vi "MIME TIFF Parser.vi"() -> ()   [LabVIEW 2014]
panel:
  out "Cluster":T1
  in  "Path":path
  out "Decompress":bool
  out "data out":string
  out "Width":u32
  out "Height":u32
  in  "error in (no error)":errorcluster
  out "error out":errorcluster
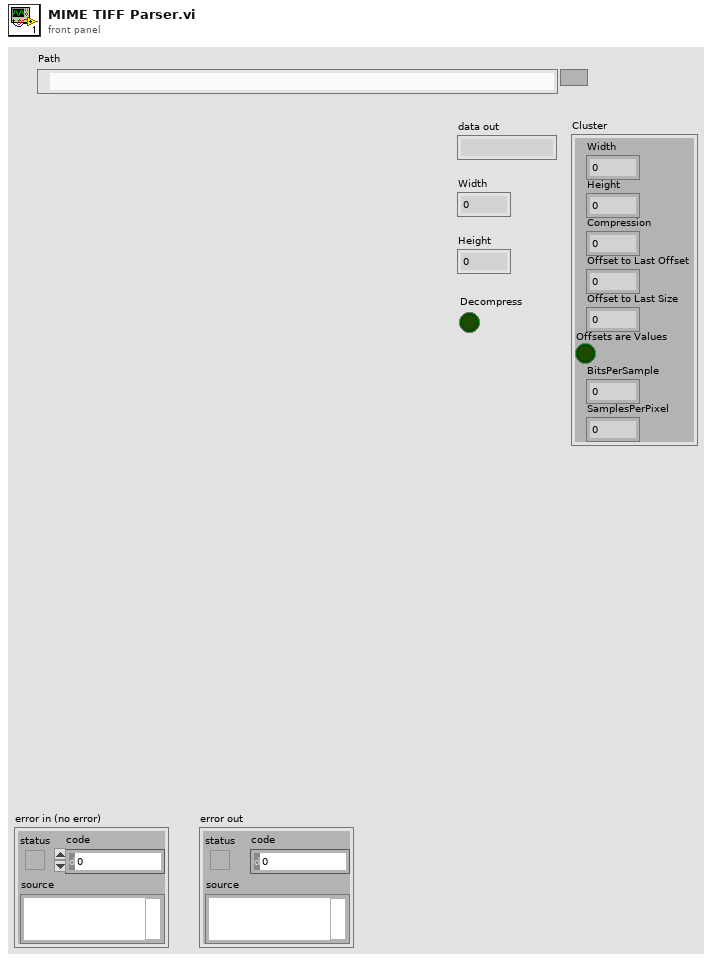
[diagram p1: front panel]
types:
  T1 = cluster{"Width":u32, "Height":u32, "Compression":u32, "Offset to Last Offset":u32, "Offset to Last Size":u32, "Offsets are Values":bool, "BitsPerSample":u32, "SamplesPerPixel":u32}
  T2 = cluster{"Tag":u16, "Type":enum16{"NONE", "Byte", "ASCII", "Short", "Long", "Rational", "SByte", "Undefined", "SShort", "SLong", "SRational", "Float", "Double"}, "Count":u32, "Value/Offset":u32}
  T3 = enum16{"big-endian, network order", "native, host order", "little-endian"}
  T4 = cluster{"Tag":u16, "Type":enum16{"NONE", "Byte", "ASCII", "Short", "Long", "Rational", "SByte", "Undefined", "SShort", "SLong", "SRational", "Float", "Double"}, "Count":u32, "Value/Offset":u32}[]
  T5 = enum16{"NONE", "Byte", "ASCII", "Short", "Long", "Rational", "SByte", "Undefined", "SShort", "SLong", "SRational", "Float", "Double"}
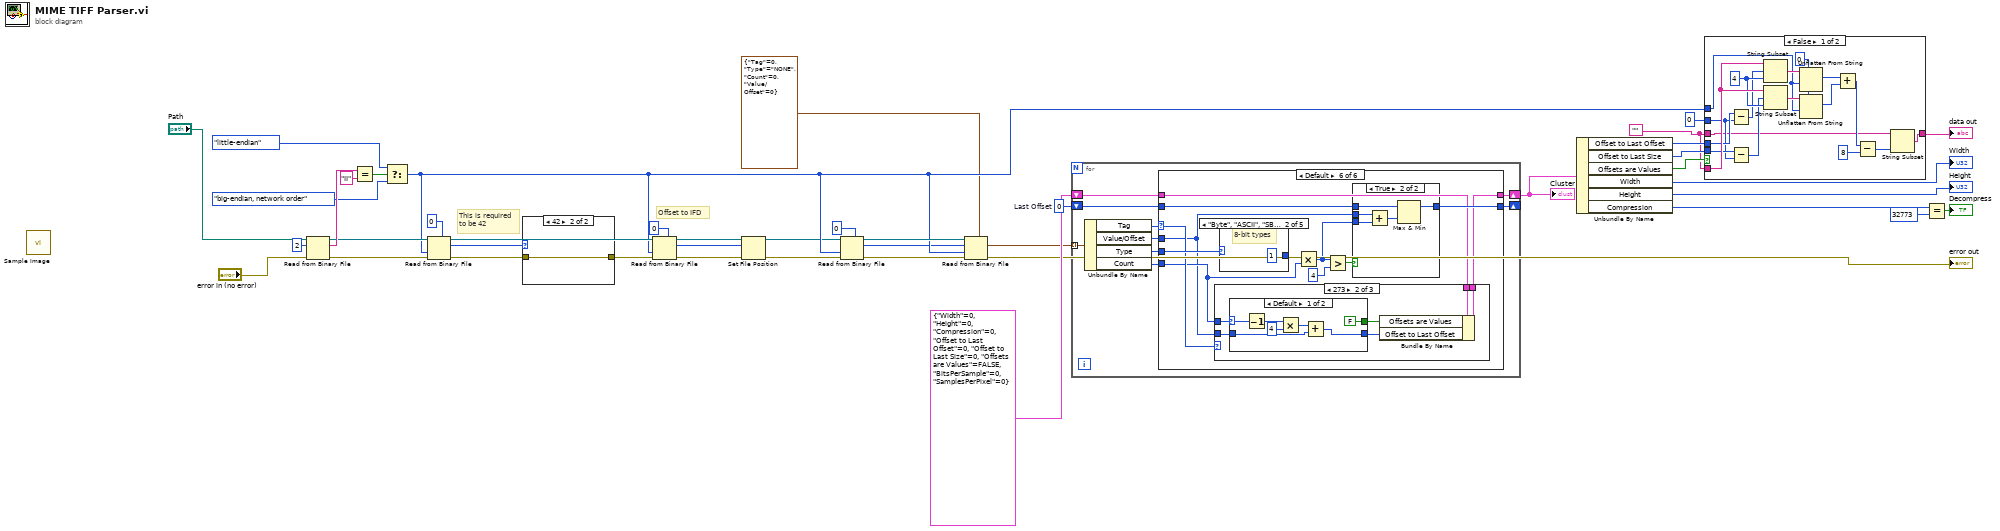
[diagram p0: block diagram]
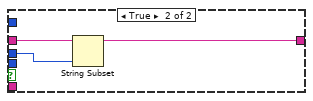
[diagram p2: hidden frame]
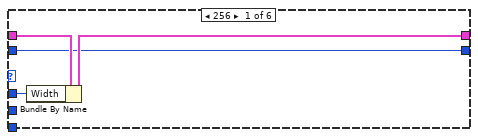
[diagram p3: hidden frame]
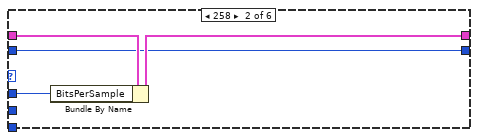
[diagram p4: hidden frame]
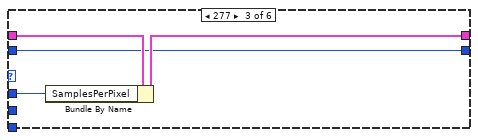
[diagram p5: hidden frame]
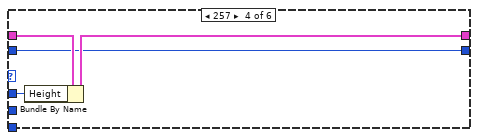
[diagram p6: hidden frame]
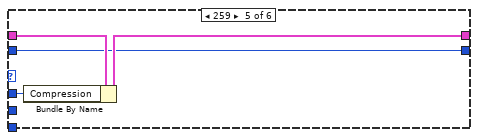
[diagram p7: hidden frame]
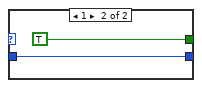
[diagram p9: hidden frame]
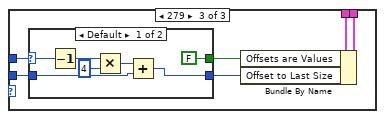
[diagram p10: hidden frame]
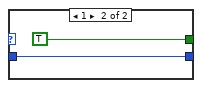
[diagram p11: hidden frame]
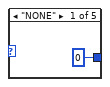
[diagram p13: hidden frame]
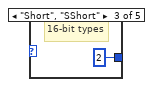
[diagram p14: hidden frame]
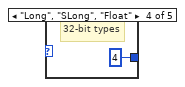
[diagram p15: hidden frame]
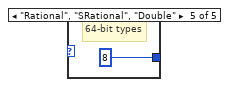
[diagram p16: hidden frame]
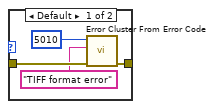
[diagram p17: hidden frame]
diagram:
  w1 = ""
  w36 = u32 0  # Last Offset
  # "Offset to IFD"
  # "This is required\nto be 42"
  n1 = call "Sample Image.vi"() -> ()  [unwired: 11 in, 1 out]
  n2 = Read from Binary File(8:"error in (no error)", 10:2 ("bytes to read"), 11:"Path") -> (0:w27:errorcluster, 2:w25:string, 3:w22:refnum<file>)  [unwired: 3 in, 1 out]
  n3 = Equal?(x=w25, y="II") -> (x = y?=w41:bool)
  n4 = Select(t=T3."little-endian" ("byte order (0:big-endian, network order)"), s=w41, f=T3."big-endian, network order" ("byte order (0:big-endian, network order)")) -> (s? t:f=w15:T3)
  n5 = Read from Binary File(5:u16 0, 8:w27, 9:w15, 11:w22) -> (0:w20:errorcluster, 2:w19:u16, 3:w43:refnum<file>)  [unwired: 2 in, 1 out]
  n6 = case shown="42" w19 {
    tunnel: w20 -> [w47 w48]
    tunnel: [w44 w48] -> w39
    frame Default {
      n7 = call <vilib>:"Error Cluster From Error Code.vi"("error in (no error)"=w47, "error message (\"\")"="TIFF format error" ("error message (\"\")"), "error code (0)"=5010) -> ("error out"=w44:errorcluster)  [unwired: 6 in]
    }
    frame 42 {
    }
  }
  n8 = Read from Binary File(5:u32 0, 8:w39, 9:w15, 11:w43) -> (0:w6:errorcluster, 2:w4:u32, 3:w8:refnum<file>)  [unwired: 2 in, 1 out]
  n9 = Set File Position(offset (in bytes) (0)=w4, refnum=w8, error in=w6) -> (refnum out=w7:refnum<file>, error out=w5:errorcluster)  [unwired: 1 in]
  n10 = Read from Binary File(5:u16 0, 8:w5, 9:w15, 11:w7) -> (0:w16:errorcluster, 2:w14:u16, 3:w38:refnum<file>)  [unwired: 2 in, 1 out]
  n11 = Read from Binary File(5:T2 {"Tag"=0, "Type"=enum."NONE", "Count"=0, "Value/Offset"=0}, 8:w16, 9:w15, 10:w14, 11:w38) -> (0:→"error out":errorcluster, 2:w13:T4)  [unwired: 1 in, 2 out]
  n12 = for {
    tunnel: w13 -> [w49] mode=indexing
    shift-right: [w55] -> w32
    shift-left: T1 {"Width"=0, "Height"=0, "Compression"=0, "Offset to Last Offset"=0, "Offset to Last Size"=0, "Offsets are Values"=FALSE, "BitsPerSample"=0, "SamplesPerPixel"=0} -> [w56]
    shift-right: [w50] -> _
    shift-left: w36 -> [w51]
    n13 = Unbundle By Name(w49) -> ("Tag"=w57:u16, "Value/Offset"=w54:u32, "Type"=w53:T5, "Count"=w52:u32)
    n14 = case shown="Default" w57 {
      selector: w57 -> [_ _ _ _ _ w82]
      tunnel: w56 -> [w61 w65 w69 w73 w77 w80]
      tunnel: [w60 w64 w68 w72 w76 w79] -> w55
      tunnel: w54 -> [w59 w63 w67 w71 w75 w78]
      tunnel: w53 -> [_ _ _ _ _ w89]
      tunnel: w52 -> [_ _ _ _ _ w81]
      tunnel: w51 -> [w58 w62 w66 w70 w74 w85]
      tunnel: [w58 w62 w66 w70 w74 w83] -> w50
      frame 256 {
        n15 = Bundle By Name(cluster=w61, "Width"=w59) -> (w60:T1)
      }
      frame 258 {
        n16 = Bundle By Name(cluster=w65, "BitsPerSample"=w63) -> (w64:T1)
      }
      frame 277 {
        n17 = Bundle By Name(cluster=w69, "SamplesPerPixel"=w67) -> (w68:T1)
      }
      frame 257 {
        n18 = Bundle By Name(cluster=w73, "Height"=w71) -> (w72:T1)
      }
      frame 259 {
        n19 = Bundle By Name(cluster=w77, "Compression"=w75) -> (w76:T1)
      }
      frame Default {
        n20 = case shown="273" w82 {
          tunnel: w81 -> [_ w94 w109]
          tunnel: w80 -> [w90 w96 w111]
          tunnel: [w90 w95 w110] -> w79
          tunnel: w78 -> [_ w91 w106]
          frame Default {
          }
          frame 273 {
            n21 = case shown="Default" w94 {
              selector: w94 -> [w103 _]
              tunnel: [FALSE TRUE] -> w93
              tunnel: [w97 w104] -> w92
              tunnel: w91 -> [w98 w104]
              frame Default {
                n22 = Decrement(x=w103) -> (x-1=w102:u32)
                n23 = Multiply(x=w102, y=u32 4) -> (x*y=w99:u32)
                n24 = Add(x=w99, y=w98) -> (x+y=w97:u32)
              }
              frame 1 {
              }
            }
            n25 = Bundle By Name(cluster=w96, "Offsets are Values"=w93, "Offset to Last Offset"=w92) -> (w95:T1)
          }
          frame 279 {
            n26 = case shown="Default" w109 {
              selector: w109 -> [w118 _]
              tunnel: [FALSE TRUE] -> w108
              tunnel: [w112 w119] -> w107
              tunnel: w106 -> [w113 w119]
              frame Default {
                n27 = Decrement(x=w118) -> (x-1=w117:u32)
                n28 = Multiply(x=w117, y=u32 4) -> (x*y=w114:u32)
                n29 = Add(x=w114, y=w113) -> (x+y=w112:u32)
              }
              frame 1 {
              }
            }
            n30 = Bundle By Name(cluster=w111, "Offsets are Values"=w108, "Offset to Last Size"=w107) -> (w110:T1)
          }
        }
        n31 = case shown="\"Byte\", \"ASCII\", \"SByte\", \"Undefined\"" w89 {
          tunnel: [0 1 2 4 8] -> w88
          frame "NONE" {
          }
          frame "Byte", "ASCII", "SByte", "Undefined" {
            # "8-bit types"
          }
          frame "Short", "SShort" {
            # "16-bit types"
          }
          frame "Long", "SLong", "Float" {
            # "32-bit types"
          }
          frame "Rational", "SRational", "Double" {
            # "64-bit types"
          }
        }
        n32 = Multiply(x=w88, y=w81) -> (x*y=w84:u32)
        n33 = Greater?(x=w84, y=u32 4) -> (0:w86:bool)
        n34 = case shown="True" w86 {
          tunnel: w78 -> [_ w126]
          tunnel: w85 -> [w121 w123]
          tunnel: w84 -> [_ w125]
          tunnel: [w121 w122] -> w83
          frame False {
          }
          frame True {
            n35 = Add(x=w126, y=w125) -> (x+y=w124:u32)
            n36 = Max & Min(x=w123, y=w124) -> (max(x,y)=w122:u32)  [unwired: 1 out]
          }
        }
      }
    }
  }
  "Cluster" <- w32
  n37 = Unbundle By Name(w32) -> ("Offset to Last Offset"=w30:u32, "Offset to Last Size"=w29:u32, "Offsets are Values"=w31:bool, "Width"=→"Width":u32, "Height"=→"Height":u32, "Compression"=w35:u32)
  n38 = case shown="False" w31 {
    tunnel: [w140 w151] -> w11
    tunnel: w1 -> [w134 w152]
    tunnel: w30 -> [w147 w150]
    tunnel: w29 -> [w146 _]
    tunnel: w1 -> [w149 _]
    tunnel: 0 -> [w145 _]
    tunnel: w15 -> [w138 _]
    frame False {
      w139 = u32 0
      w148 = 4 ("length (rest)")
      n39 = Subtract(x=w147, y=w145) -> (x-y=w144:u32)
      n40 = Subtract(x=w146, y=w145) -> (x-y=w143:u32)
      n41 = String Subset(string=w149, offset (0)=w144, length (rest)=w148) -> (substring=w142:string)
      n42 = String Subset(string=w149, offset (0)=w143, length (rest)=w148) -> (substring=w141:string)
      n43 = Unflatten From String(type=w139, binary string=w142, byte order (0:big-endian, network order)=w138) -> (value=w137:u32)  [unwired: 2 in, 2 out]
      n44 = Unflatten From String(type=w139, binary string=w141, byte order (0:big-endian, network order)=w138) -> (value=w136:u32)  [unwired: 2 in, 2 out]
      n45 = Add(x=w137, y=w136) -> (x+y=w135:u32)
      n46 = Subtract(x=w135, y=u32 8) -> (x-y=w133:u32)
      n47 = String Subset(string=w134, length (rest)=w133) -> (substring=w140:string)  [unwired: 1 in]
    }
    frame True {
      n48 = String Subset(string=w152, length (rest)=w150) -> (substring=w151:string)  [unwired: 1 in]
    }
  }
  "data out" <- w11
  n49 = Equal?(x=w35, y=u32 32773) -> (x = y?=→"Decompress":bool)
